vi "Steering PID.vi"(0 "steeringSetpoints":dbl[](array[numeric])) -> (1 "invertPower":bool[](array[boolean]), 2 "steeringPower":dbl[](array[numeric]))   [LabVIEW 2019]
uses:
  swerveData.vi
  <vilib>/addons/control/pid/pid.llb/PID (DBL).vi
  <vilib>/addons/control/pid/pid.llb/PID Output Rate Limiter (DBL).vi
  <vilib>/addons/control/pid/NI_PID_pid.lvlib
panel:
  in  "PID gains":T1={"proportional gain (Kc)"=3.7, "integral time (Ti, min)"=0.0, "derivative time (Td, min)"=0.5}
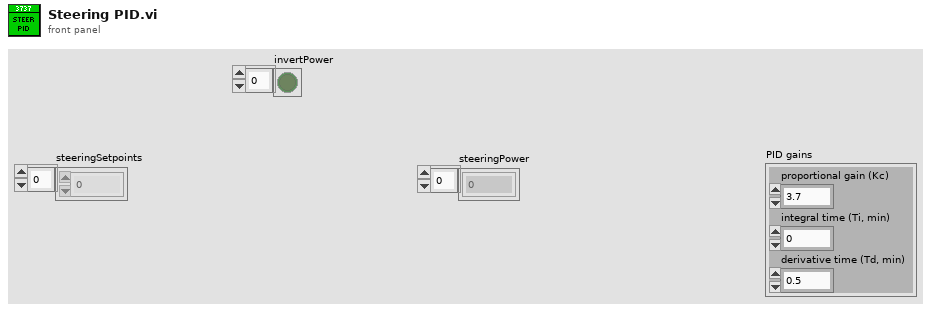
[diagram p1: front panel]
types:
  T1 = cluster{"proportional gain (Kc)":dbl, "integral time (Ti, min)":dbl, "derivative time (Td, min)":dbl}
  T2 = cluster{"[0]":dbl, "[1]":dbl, "[2]":dbl, "[3]":dbl, "[4]":dbl, "[5]":dbl, "[6]":dbl, "[7]":dbl, "[8]":dbl}
  T3 = cluster{"output":dbl, "output":dbl, "output":dbl, "output":dbl}
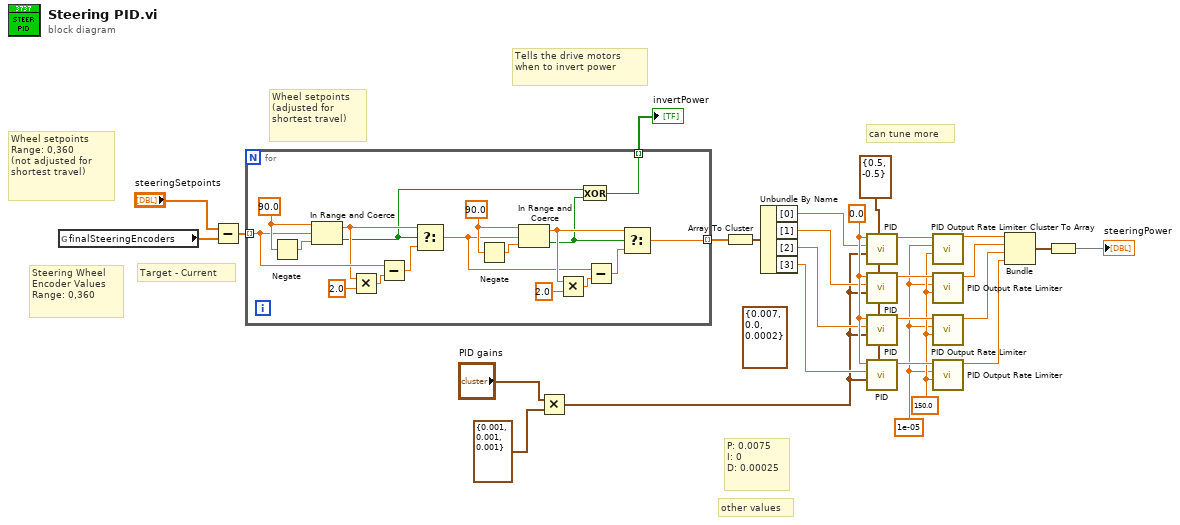
[diagram p0: block diagram]
diagram:
  w11 = 0.0 ("setpoint")
  w12 = cluster{"output high":dbl, "output low":dbl} {"output high"=0.5, "output low"=-0.5} ("output range")
  (unwired) T1 {"proportional gain (Kc)"=0.007, "integral time (Ti, min)"=0.0, "derivative time (Td, min)"=0.0002} ("PID gains")
  w10 = 150.0 ("initial output")
  w9 = 1e-05 ("initial output")
  # "can tune more"
  # "other values"
  # "P: 0.0075\nI: 0\nD: 0.00025"
  # "Steering Wheel\nEncoder Values\nRange: 0,360"
  # "Wheel setpoints\n(adjusted for \nshortest travel)"
  # "Target - Current"
  # "Wheel setpoints\nRange: 0,360\n(not adjusted for \nshortest travel)"
  # "Tells the drive motors when to invert power"
  n1 = global read "swerveData.vi" "finalSteeringEncoders"() -> (w26:dbl[])
  n2 = Subtract(x="steeringSetpoints", y=w26) -> (x-y=w27:dbl[])
  n3 = for {
    tunnel: w27 -> [w43] mode=indexing
    tunnel: [w29] -> w1 mode=indexing
    tunnel: [w28] -> w23 mode=indexing
    w33 = 90.0
    w45 = 90.0
    n4 = Negate(x=w45) -> (-x=w44:dbl)
    n5 = In Range and Coerce(upper limit=w45, x=w43, lower limit=w44) -> (coerced(x)=w40:dbl, In Range?=w30:bool)
    n6 = Multiply(x=w40, y=2.0) -> (x*y=w41:dbl)
    n7 = Subtract(x=w43, y=w41) -> (x-y=w42:dbl)
    n8 = Select(t=w40, s=w30, f=w42) -> (s? t:f=w32:dbl)
    n9 = Negate(x=w33) -> (-x=w34:dbl)
    n10 = In Range and Coerce(upper limit=w33, x=w32, lower limit=w34) -> (coerced(x)=w37:dbl, In Range?=w31:bool)
    n11 = Multiply(x=w37, y=2.0) -> (x*y=w36:dbl)
    n12 = Exclusive Or(1:w31, 2:w30) -> (0:w29:bool)
    n13 = Subtract(x=w32, y=w36) -> (x-y=w35:dbl)
    n14 = Select(t=w37, s=w31, f=w35) -> (s? t:f=w28:dbl)
  }
  "invertPower" <- w1
  n15 = Multiply(x="PID gains", y=T1 {"proportional gain (Kc)"=0.001, "integral time (Ti, min)"=0.001, "derivative time (Td, min)"=0.001}) -> (x*y=w2:T1)
  n16 = Array To Cluster(array=w23) -> (cluster=w22:T2)
  n17 = Unbundle By Name(w22) -> ("[0]"=w5:dbl, "[1]"=w6:dbl, "[2]"=w7:dbl, "[3]"=w8:dbl)
  n18 = call-poly <vilib>:"PID.vi"("output range"=w12, "PID gains"=w2, "process variable"=w5, "setpoint"=w11) -> ("output"=w24:dbl)  [unwired: 6 in, 1 out]
  n19 = call-poly <vilib>:"PID.vi"("output range"=w12, "PID gains"=w2, "process variable"=w6, "setpoint"=w11) -> ("output"=w21:dbl)  [unwired: 6 in, 1 out]
  n20 = call-poly <vilib>:"PID.vi"("output range"=w12, "PID gains"=w2, "process variable"=w7, "setpoint"=w11) -> ("output"=w20:dbl)  [unwired: 6 in, 1 out]
  n21 = call-poly <vilib>:"PID.vi"("output range"=w12, "PID gains"=w2, "process variable"=w8, "setpoint"=w11) -> ("output"=w19:dbl)  [unwired: 6 in, 1 out]
  n22 = call-poly <vilib>:"PID Output Rate Limiter.vi"("output rate (EGU/min)"=w10, "initial output"=w9, "input (controller output)"=w24) -> ("output"=w15:dbl)  [unwired: 5 in, 1 out]
  n23 = call-poly <vilib>:"PID Output Rate Limiter.vi"("output rate (EGU/min)"=w10, "initial output"=w9, "input (controller output)"=w21) -> ("output"=w14:dbl)  [unwired: 5 in, 1 out]
  n24 = call-poly <vilib>:"PID Output Rate Limiter.vi"("output rate (EGU/min)"=w10, "initial output"=w9, "input (controller output)"=w20) -> ("output"=w16:dbl)  [unwired: 5 in, 1 out]
  n25 = call-poly <vilib>:"PID Output Rate Limiter.vi"("output rate (EGU/min)"=w10, "initial output"=w9, "input (controller output)"=w19) -> ("output"=w17:dbl)  [unwired: 5 in, 1 out]
  n26 = Bundle("output"=w15, "output"=w14, "output"=w16, "output"=w17) -> (w18:T3)  [unwired: 1 in]
  n27 = Cluster To Array(cluster=w18) -> (array=→"steeringPower":dbl[])
